vi "PIDSwerveSpeed.vi"() -> ()   [LabVIEW 2010]
panel:
  in  "PID Swerve Speed":dbl
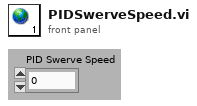
[diagram p1: front panel]
diagram:
